vi "Example PDC Reader.vi"(8 "error in (no error)":errorcluster) -> (0 "error out":errorcluster)   [LabVIEW 2013]
doc: "Use this template to build a producer/consumer design pattern with events to produce queue items. Use this design pattern instead of the User Interface Event Handler pattern for user interfaces when you want to execute code asynchronously in response to an event without slowing the user interface responsiveness."
uses:
  <vilib>/platform/TimedLoop/XDataNode/XDataNode.xnode
  <vilib>/Platform/TimedLoop/XDataNode/timing_clust.ctl
  <vilib>/Platform/TimedLoop/XDataNode/XDNodeRunTimeDep.lvlib
  <vilib>/Platform/TimedLoop/XDataNode/wakeup.ctl
  <vilib>/Platform/TimedLoop/XDataNode/nitl_modes.ctl
  PMU Recorder Light/PMU Recorder Light.lvlib
panel:
  out "Waveform Chart":waveform(sgl)(graph)
  out "Digital Signals":bool[][](array[boolean])
  out "Phasor Signals":csg[][](array[numeric])
  out "Error":bool
  out "Status Loop":bool
  out "Timed Loop":bool
  out "Execution Loop":bool
  out "Event Loop":bool
  out "Has New Data?":bool
  out "Analog Signals":sgl[][](array[numeric])
  out "Timestamp":timestamp[](array[timestamp])
  in  "Channel Selector":bool
  out "Connected":bool
  out "Configuration File Received":bool
  out "Buffer Active":bool
  in  "Activate PRL Read":bool=TRUE
  in  "Refresh Rate":i64(ring)=200 items=["50 Hz"=20, "20 Hz"=50, "10 Hz"=100, "5 Hz"=200, "2 Hz"=500, "1 Hz"=1000, "Every 2 sec"=2000, "Every 5 sec"=5000, "Every 10 sec"=10000, "Every minute"=60000]
  out "Quitting":bool
  in  "Quit":bool
  in  "PRL Visible":bool
  out "Status":string
  # "INPUT"
  # "INTERMEDIATE"
  # "OUTPUT"
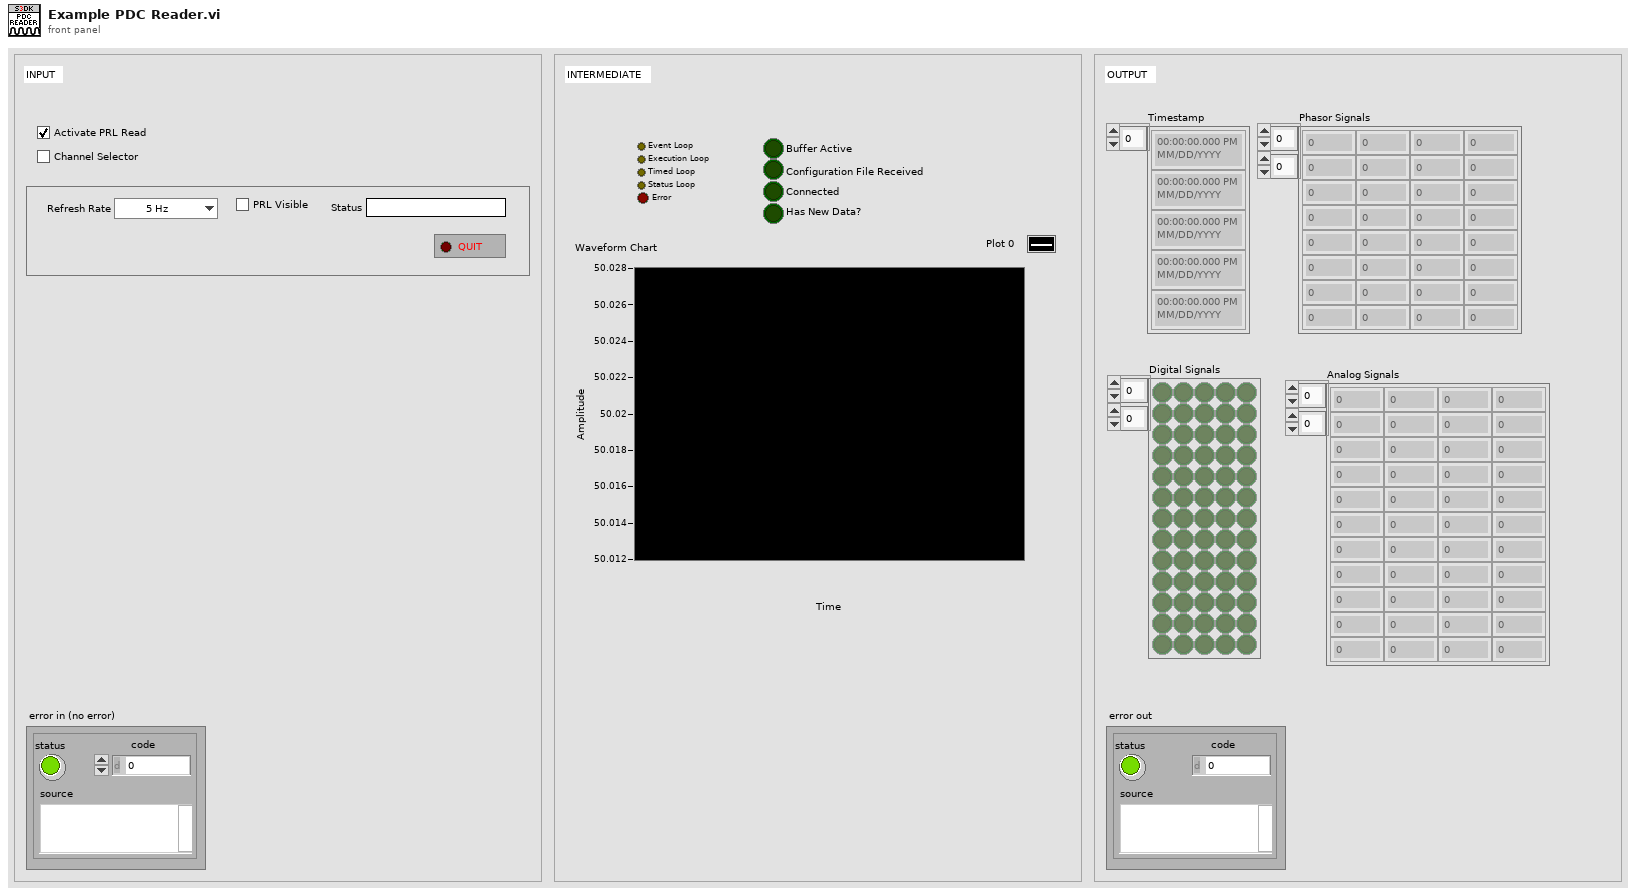
[diagram p1: front panel]
types:
  T1 = enum16{"Run", "Startup", "Get Status", "Pause", "Continue", "Shutdown", "Abort", "Open Panel", "Close Panel"}
  T2 = enum32{"Invalid", "Standard", "Closed", "Hidden", "Minimized", "Maximized"}
  T3 = typedef "XDNodeRunTimeDep.lvlib/timing_clust.ctl" = cluster{"Expected End [f-1]":u64, "Actual End [f-1]":u64, "Finished Late? [f-1]":bool, "Expected End [i-1]":u64, "Actual End [i-1]":u64, "Finished Late? [i-1]":bool, "Expected Start [i]":u64, "Actual Start [i]":u64, "Expected Start [f]":u64, "Actual Start [f]":u64, "Source Name":string, "Structure Name":string, "Period":i64, "Deadline":i64, "Offset":i64, "Start":i64, "Priority":i32, "Timeout":i32, "Mode":T4, "Wakeup Reason":T5, "Error":errorcluster, "Source Type":string, "Secondary Source Type":string, "Global End Time":u64, "Global Start Time":u64, "Frame Duration":u64, "Iteration Duration":u64, "Assigned CPU":i32, "I/O Scan Engine Mode":u32}
  T4 = typedef "XDNodeRunTimeDep.lvlib/nitl_modes.ctl" = enum32{"No Change", "Process missed periods, maintain original phase", "Discard missed periods, maintain original phase", "Process missed periods, ignore original phase", "Discard missed periods, ignore original phase"}
  T5 = typedef "XDNodeRunTimeDep.lvlib/wakeup.ctl" = enum32{"Normal", "Aborted", "Asynchronous wakeup", "Timing source error", "Timed loop error", "Timeout"}
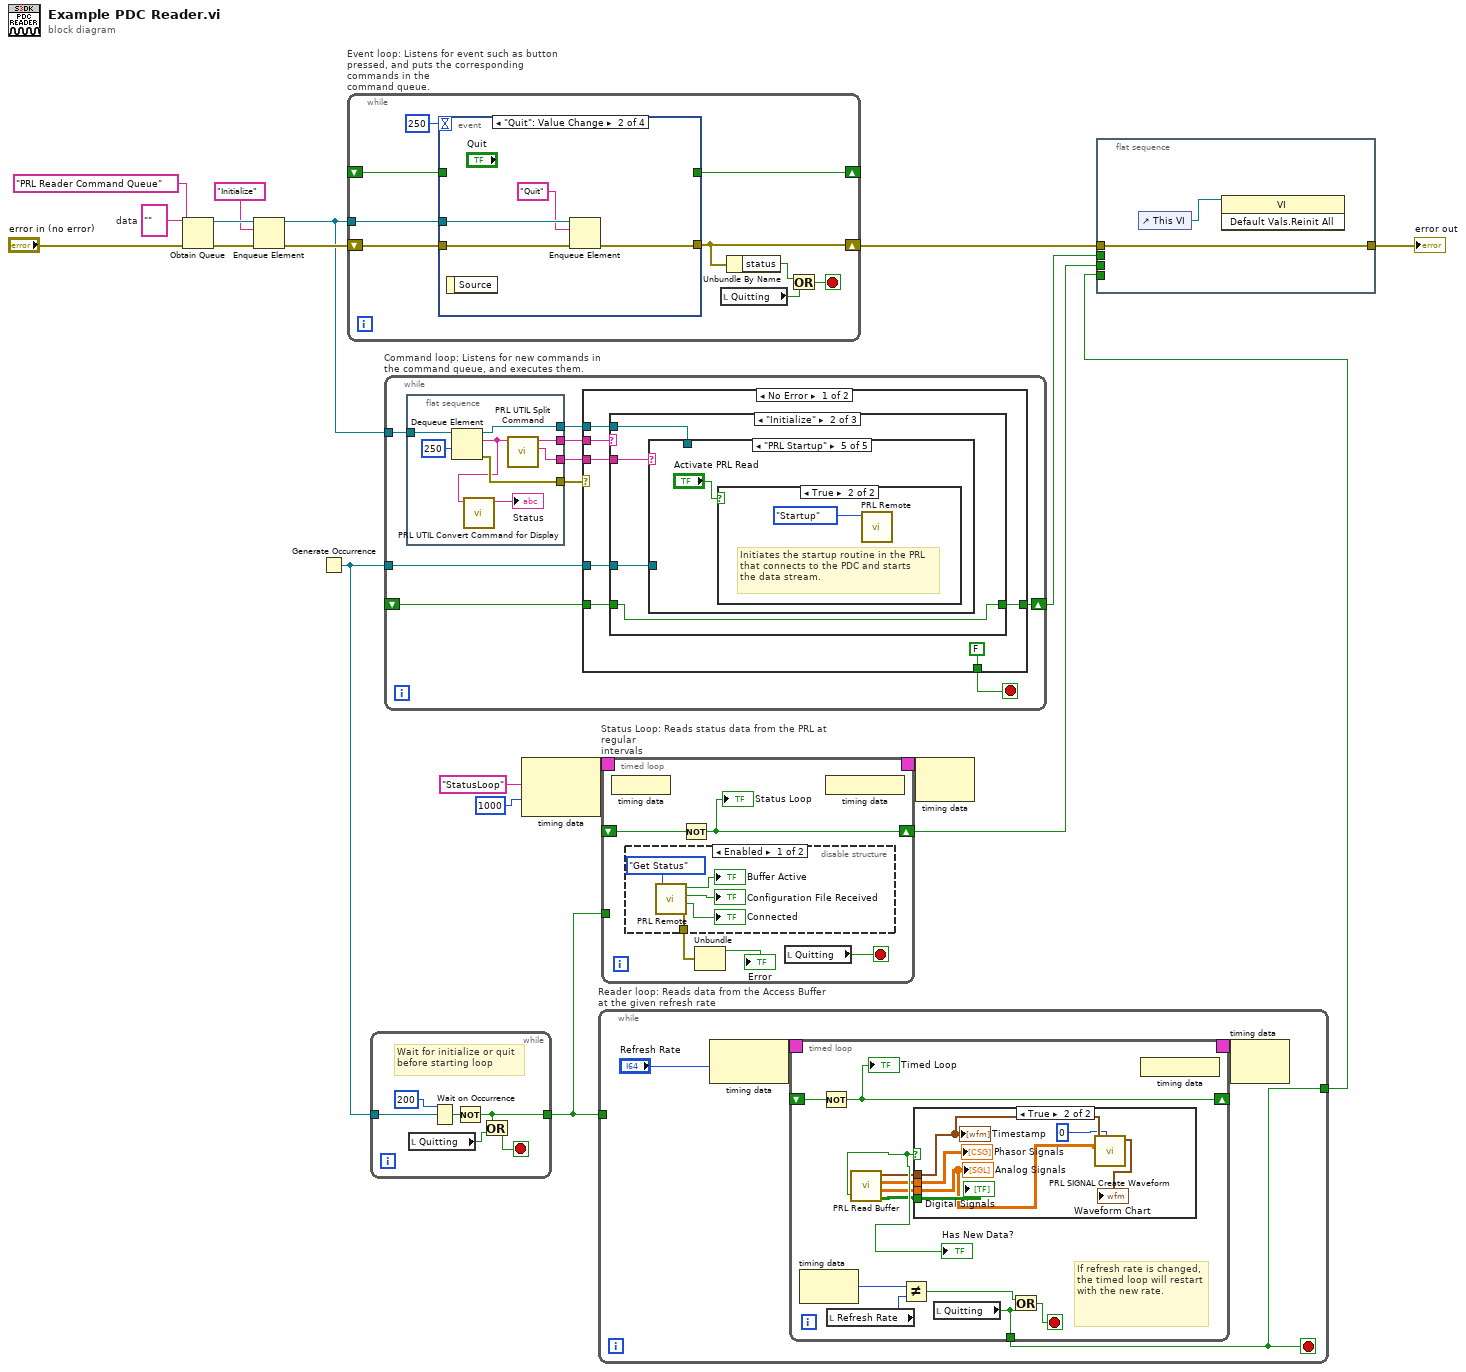
[diagram p0: block diagram]
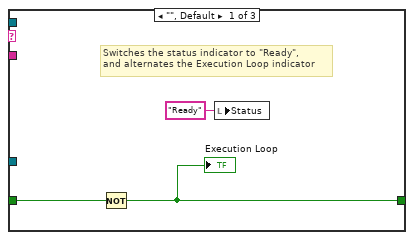
[diagram p4: hidden frame]
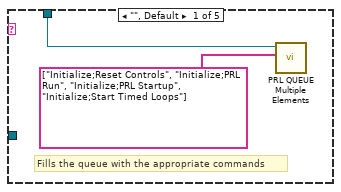
[diagram p5: hidden frame]
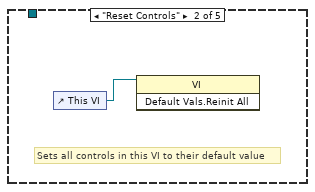
[diagram p6: hidden frame]
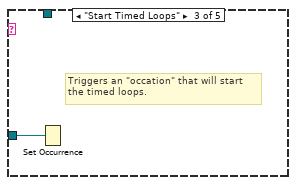
[diagram p7: hidden frame]
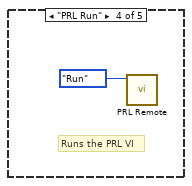
[diagram p8: hidden frame]
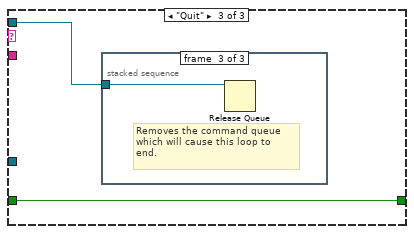
[diagram p10: hidden frame]
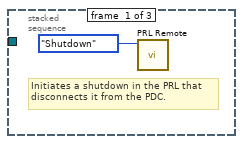
[diagram p11: hidden frame]
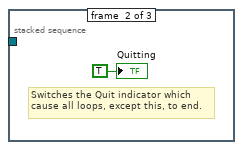
[diagram p12: hidden frame]
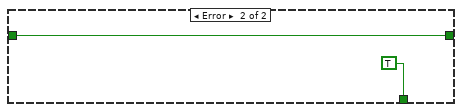
[diagram p13: hidden frame]
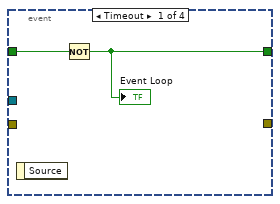
[diagram p14: hidden frame]
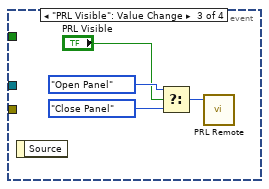
[diagram p15: hidden frame]
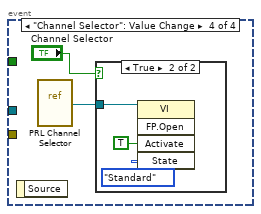
[diagram p16: hidden frame]
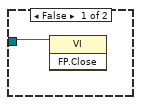
[diagram p17: hidden frame]
diagram:
  w19 = ""  # data
  n1 = Obtain Queue(name (unnamed)="PRL Reader Command Queue", element data type=w19, error in (no error)="error in (no error)") -> (queue out=w18:refnum<queue>, error out=w17:errorcluster)  [unwired: 2 in, 1 out]
  n2 = Enqueue Element(queue=w18, element="Initialize", error in (no error)=w17) -> (queue out=w11:refnum<queue>, error out=w16:errorcluster)  [unwired: 1 in, 1 out]
  n3 = Generate Occurrence() -> (w14:refnum<k4>)
  n4 = while "Event loop: Listens for event such as button pressed, and puts the corresponding commands in the\ncommand queue." {
    shift-right: [w25] -> w6
    shift-left: w16 -> [w27]
    tunnel: w11 -> [w28]
    shift-right: [w20] -> _
    shift-left: _ -> [w21]
    stop <- w26 stop-if-true
    n5 = event shown="[1] \"Quit\": Value Change" {
      selector: _ -> [_ _ _ _]
      dyn-events: _ -> [_ _ _ _]
      timeout: 250 -> [_ _ _ _]
      tunnel: w28 -> [_ w33 _ _]
      tunnel: w27 -> [_ w34 _ _]
      tunnel: [_ w32 _ _] -> w25
      tunnel: w21 -> [w30 _ _ _]
      tunnel: [w29 _ _ _] -> w20
      event Timeout {
        n6 = event-data() -> ()  [unwired: 1 in, 1 out]
        n7 = Not(x=w30) -> (.not. x?=w29:bool)
        "Event Loop" <- w29
      }
      event "Quit": Value Change {
        n8 = event-data() -> ()  [unwired: 1 in, 1 out]
        n9 = Enqueue Element(queue=w33, element="Quit", error in (no error)=w34) -> (error out=w32:errorcluster)  [unwired: 1 in, 2 out]
      }
      event "PRL Visible": Value Change {
        n10 = event-data() -> ()  [unwired: 1 in, 1 out]
        n11 = Select(t=T1."Open Panel" ("Action"), s="PRL Visible", f=T1."Close Panel" ("Action")) -> (s? t:f=w35:T1)
        n12 = call "PRL Remote.vi"("Action"=w35) -> ()  [unwired: 5 in, 6 out]
      }
      event "Channel Selector": Value Change {
        n13 = event-data() -> ()  [unwired: 1 in, 1 out]
        n14 = vi-ref "PRL Channel Selector.vi"() -> (w40:refnum<vi>)
        n15 = case shown="True" "Channel Selector" {
          tunnel: w40 -> [w41 w44]
          frame False {
            n16 = invoke class="VI" method="FP.Close"(reference=w41) -> ()  [unwired: 2 in, 3 out]
          }
          frame True {
            n17 = invoke class="VI" method="FP.Open"(reference=w44, "Activate"=TRUE ("Activate?"), "State"=T2."Standard") -> ()  [unwired: 2 in, 5 out]
          }
        }
      }
    }
    n18 = local read "Quitting"() -> (w22:bool)
    n19 = Unbundle By Name(w25) -> ("status"=w24:bool)
    n20 = Or(x=w24, y=w22) -> (x .or. y?=w26:bool)
  }
  n21 = while {
    tunnel: w14 -> [w50]
    tunnel: [w45] -> w8
    stop <- w46 stop-if-true
    # "Wait for initialize or quit\nbefore starting loop"
    n22 = local read "Quitting"() -> (w47:bool)
    n23 = Wait on Occurrence(2:w50, 3:200 ("ms timeout (-1)")) -> (0:w48:bool)  [unwired: 1 in]
    n24 = Not(x=w48) -> (.not. x?=w45:bool)
    n25 = Or(x=w45, y=w47) -> (x .or. y?=w46:bool)
  }
  n26 = while "Command loop: Listens for new commands in the command queue, and executes them." {
    tunnel: w11 -> [w59]
    tunnel: w14 -> [w56]
    shift-right: [w51] -> w5
    shift-left: _ -> [w52]
    stop <- w54 stop-if-true
    n27 = flat-sequence {
      tunnel: w59 -> [w67]
      tunnel: [w66] -> w58
      tunnel: [w65] -> w57
      tunnel: [w63] -> w55
      tunnel: [w60] -> w53
      frame #0 {
        n28 = Dequeue Element(queue=w67, timeout in ms (-1)=250) -> (queue out=w65:refnum<queue>, element=w62:string, error out=w66:errorcluster)  [unwired: 1 in, 1 out]
        n29 = call "PRL UTIL Convert Command for Display.vi"("Command In"=w62) -> ("Command Out"=→"Status":string)  [unwired: 10 in]
        n30 = call "PRL UTIL Split Command.vi"("Command"=w62) -> ("Parameters"=w60:string, "Command Out"=w63:string)  [unwired: 9 in]
      }
    }
    n31 = case shown="No Error" w58 {
      tunnel: w55 -> [w74 _]
      tunnel: w57 -> [w73 _]
      tunnel: w56 -> [w72 _]
      tunnel: [FALSE TRUE] -> w54
      tunnel: w53 -> [w70 _]
      tunnel: w52 -> [w69 w94]
      tunnel: [w68 w94] -> w51
      frame No Error {
        n32 = case shown="\"Initialize\"" w74 {
          tunnel: w73 -> [_ w80 w89]
          tunnel: w72 -> [_ w79 _]
          tunnel: w70 -> [_ w81 _]
          tunnel: w69 -> [w76 w78 w90]
          tunnel: [w75 w78 w90] -> w68
          frame "", Default {
            # "Switches the status indicator to \"Ready\",\nand alternates the Execution Loop indicator"
            n33 = Not(x=w76) -> (.not. x?=w75:bool)
            "Execution Loop" <- w75
            n34 = local write "Status"("Ready" ("Status")) -> ()
          }
          frame "Initialize" {
            n35 = case shown="\"PRL Startup\"" w81 {
              tunnel: w80 -> [w83 _ _ _ _]
              tunnel: w79 -> [_ _ w85 _ _]
              frame "", Default {
                # "Fills the queue with the appropriate commands"
                n36 = call "PRL QUEUE Multiple Elements.vi"("Elements to Add"=string[] ["Initialize;Reset Controls", "Initialize;PRL Run", "Initialize;PRL Startup", "Initialize;Start Timed Loops"], "queue"=w83) -> ()  [unwired: 8 in, 2 out]
              }
              frame "Reset Controls" {
                # "Sets all controls in this VI to their default value"
                n37 = control-ref of="This VI"() -> (w84:refnum<vi>)
                n38 = invoke class="VI" method="Default Vals.Reinit All"(reference=w84) -> ()  [unwired: 2 in, 3 out]
              }
              frame "Start Timed Loops" {
                # "Triggers an \"occation\" that will start \nthe timed loops."
                n39 = Set Occurrence(w85) -> ()
              }
              frame "PRL Run" {
                # "Runs the PRL VI"
                n40 = call "PRL Remote.vi"("Action"=T1."Run") -> ()  [unwired: 5 in, 6 out]
              }
              frame "PRL Startup" {
                n41 = case shown="True" "Activate PRL Read" {
                  frame False {
                  }
                  frame True {
                    # "Initiates the startup routine in the PRL\nthat connects to the PDC and starts\nthe data stream."
                    n42 = call "PRL Remote.vi"("Action"=T1."Startup") -> ()  [unwired: 5 in, 6 out]
                  }
                }
              }
            }
          }
          frame "Quit" {
            n43 = stacked-sequence {
              tunnel: w89 -> [_ _ w93]
              frame #0 {
                # "Initiates a shutdown in the PRL that\ndisconnects it from the PDC."
                n44 = call "PRL Remote.vi"("Action"=T1."Shutdown") -> ()  [unwired: 5 in, 6 out]
              }
              frame #1 {
                # "Switches the Quit indicator which\ncause all loops, except this, to end."
                "Quitting" <- TRUE ("Quitting")
              }
              frame #2 {
                # "Removes the command queue\nwhich will cause this loop to\nend."
                n45 = Release Queue(queue=w93) -> ()  [unwired: 2 in, 3 out]
              }
            }
          }
        }
      }
      frame Error {
      }
    }
  }
  n46 = node-c288("StatusLoop" ("Structure Name"), i64 1000 ("Period")) -> (w13:T3)
  n47 = while "Reader loop: Reads data from the Access Buffer at the given refresh rate" {
    tunnel: w8 -> [_]
    tunnel: [w96] -> w1
    stop <- w96 stop-if-true
    n48 = node-c288("Refresh Rate") -> (w99:T3)
    n49 = timed-loop {
      timing: w99 -> [_]
      timing-out: [_] -> w98
      tunnel: [w108] -> w96
      shift-right: [w105] -> _
      shift-left: _ -> [w106]
      stop <- w109 stop-if-true
      # "If refresh rate is changed, the timed loop will restart with the new rate."
      n50 = node-c288() -> (w111:i64)  [unwired: 1 in]
      n51 = Not(x=w106) -> (.not. x?=w105:bool)
      "Timed Loop" <- w105
      n52 = local read "Refresh Rate"() -> (w110:i64)
      n53 = call "PRL Read Buffer .vi"() -> ("Digital Signals"=w100:bool[][], "Analog Signals"=w101:sgl[][], "Phasor Signals"=w102:csg[][], "Timestamp"=w103:timestamp[], "Has Data"=w104:bool)  [unwired: 6 in, 1 out]
      "Has New Data?" <- w104
      n54 = Not Equal?(x=w111, y=w110) -> (x != y?=w107:bool)
      n55 = case shown="True" w104 {
        tunnel: w103 -> [_ w115]
        tunnel: w101 -> [_ w113]
        tunnel: w102 -> [_ w117]
        tunnel: w100 -> [_ w116]
        frame False {
        }
        frame True {
          n56 = call "PRL SIGNAL Create Waveform.vi"("Index"=0 ("index (row)"), "Analog Signals"=w113, "Timestamp"=w115) -> ("output waveform"=→"Waveform Chart":waveform(sgl))  [unwired: 8 in]
          "Timestamp" <- w115
          "Analog Signals" <- w113
          "Phasor Signals" <- w117
          "Digital Signals" <- w116
        }
      }
      n57 = local read "Quitting"() -> (w108:bool)
      n58 = Or(x=w107, y=w108) -> (x .or. y?=w109:bool)
      n59 = node-c288() -> ()  [unwired: 1 out]
    }
    n60 = node-c288(w98) -> ()  [unwired: 1 out]
  }
  n61 = timed-loop "Status Loop: Reads status data from the PRL at regular\nintervals" {
    timing: w13 -> [_]
    timing-out: [_] -> w12
    tunnel: w8 -> [_]
    shift-right: [w127] -> w4
    shift-left: _ -> [w128]
    stop <- w129 stop-if-true
    n62 = node-c288() -> ()  [unwired: 1 in]
    n63 = disable-structure shown="Enabled" {
      disable-tunnel: [w130 _] -> w126
      frame Enabled {
        n64 = call "PRL Remote.vi"("Action"=T1."Get Status") -> ("error out"=w130:errorcluster, "Connected"=→"Connected":bool, "Configuration File Received"=→"Configuration File Received":bool, "Buffer Active"=→"Buffer Active":bool)  [unwired: 5 in, 2 out]
      }
      frame Disabled {
      }
    }
    n65 = Not(x=w128) -> (.not. x?=w127:bool)
    "Status Loop" <- w127
    n66 = Unbundle(w126) -> ("status"=→"Error":bool)  [unwired: 2 out]
    n67 = local read "Quitting"() -> (w129:bool)
    n68 = node-c288() -> ()  [unwired: 1 out]
  }
  n69 = node-c288(w12) -> ()  [unwired: 1 out]
  n70 = flat-sequence {
    tunnel: w6 -> [w137]
    tunnel: w5 -> [_]
    tunnel: w4 -> [_]
    tunnel: w1 -> [_]
    tunnel: [w137] -> w2
    frame #0 {
      n71 = control-ref of="This VI"() -> (w138:refnum<vi>)
      n72 = invoke class="VI" method="Default Vals.Reinit All"(reference=w138) -> ()  [unwired: 2 in, 3 out]
    }
  }
  "error out" <- w2
